vi "SVFA Spectrum Peak Search.vi"   [LabVIEW 2017]
doc: "Performs a peak search on a spectrum or spectra. The spectrum or spectra can be in either the frequency domain or the order domain. Detects single or multiple peaks in Power, PSD, and COP spectra. Wire data to the <B>spectrum</B> input to determine the polymorphic instance to use or manually select the instance."
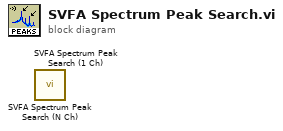
[diagram p0: block diagram]
diagram:
  n1 = call <vilib>:"SVFA Spectrum Peak Search (N Ch).vi"() -> ()  [unwired: 15 in, 5 out]
  n2 = call <vilib>:"SVFA Spectrum Peak Search (1 Ch).vi"() -> ()  [unwired: 15 in, 5 out]
